vi "TW_WriteData.vi"(6 "Type":string, 9 "value":string, 11 "Property":string) -> ()   [LabVIEW 2020]
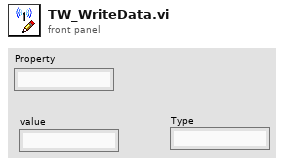
[diagram p1: front panel]
types:
  T1 = enum16{"GET", "PUT", "POST", "MultiPOST", "DELETE"}
  T2 = cluster{"Name":string, "BaseURL":string, "AppKey":string, "Headers":string[], "Timeout":i32}
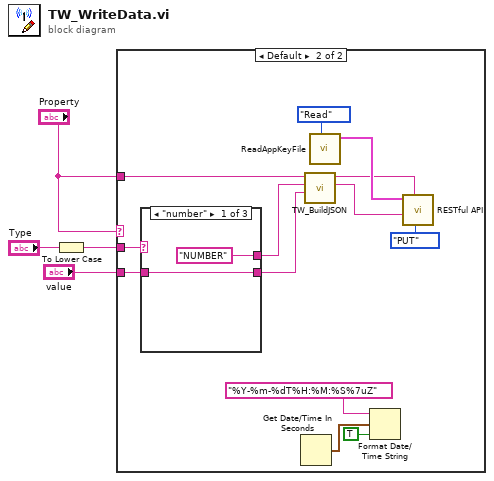
[diagram p0: block diagram]
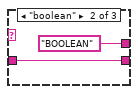
[diagram p3: hidden frame]
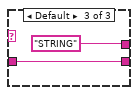
[diagram p4: hidden frame]
diagram:
  n1 = To Lower Case(string="Type") -> (all lower case string=w1:string)
  n2 = case shown="Default" "Property" {
    tunnel: "Property" -> [_ w11]
    tunnel: "value" -> [_ w5]
    tunnel: w1 -> [_ w6]
    frame "" {
    }
    frame Default {
      n3 = case shown="\"number\"" w6 {
        tunnel: ["NUMBER" ("type") "BOOLEAN" ("type") "STRING" ("type")] -> w8
        tunnel: [w18 w20 w22] -> w7
        tunnel: w5 -> [w18 w20 w22]
        frame "number" {
        }
        frame "boolean" {
        }
        frame Default {
        }
      }
      n4 = Get Date/Time In Seconds() -> (seconds since 1Jan1904=w16:timestamp)
      n5 = call "TW_BuildJSON.vi"("Value"=w7, "type"=w8, "Thingworx"=w11) -> ("JSON"=w9:string, "URL"=w10:string)  [unwired: 7 in]
      n6 = call "ReadAppKeyFile.vi"("Task"=enum16{"Read", "Write"}."Read") -> ("Device Out"=w12:T2)  [unwired: 8 in, 2 out]
      n7 = Format Date/Time String(time format string (%c)="%Y-%m-%dT%H:%M:%S%7uZ", seconds (now)=w16, UTC format=TRUE) -> ()  [unwired: 1 out]
      n8 = call "RESTful API.vi"("Method"=T1."PUT", "url"=w10, "JSON"=w9, "Device In"=w12) -> ()  [unwired: 5 in, 3 out]
    }
  }
